vi "Open.vi"(8 "error in (no error)":errorcluster, 11 "DeploySerialResource in":refnum<class "SerialResource.lvclass">) -> (0 "error out":errorcluster, 3 "DeploySerialResource out":refnum<class "SerialResource.lvclass">)   [LabVIEW 2020, in "PicoG-Core.lvlib" / "SerialResource.lvclass"]
uses:
  SerialResource.lvclass
  SerialResource.lvclass/SerialResource.ctl
  <vilib>/IlluminatedG/IG Serial Stream/Stream-Serial/Serial Client/Serial Client.lvclass
  <vilib>/IlluminatedG/IG Serial Stream/Stream-Serial/Serial Client/Stop Bits.ctl
  <vilib>/IlluminatedG/IG Serial Stream/Stream-Serial/Serial Client/Flow Control.ctl
  <vilib>/IlluminatedG/IG Serial Stream/Stream-Serial/Serial Client/Parity.ctl
  <vilib>/IlluminatedG/IG Serial Stream/Stream-Serial/Serial Client/Port Config.ctl
  <vilib>/IlluminatedG/lv-stream/Endpoint/Endpoint.lvclass
  C:/Program Files (x86)/National Instruments/LabVIEW 2020/vi.lib/IlluminatedG/lv-stream/Connection/Connection.lvclass
  C:/Program Files (x86)/National Instruments/LabVIEW 2020/vi.lib/IlluminatedG/lv-stream/Endpoint/Endpoint.lvclass
  C:/Program Files (x86)/National Instruments/LabVIEW 2020/vi.lib/IlluminatedG/IG Serial Stream/Stream-Serial/Serial Client/Serial Client.lvclass
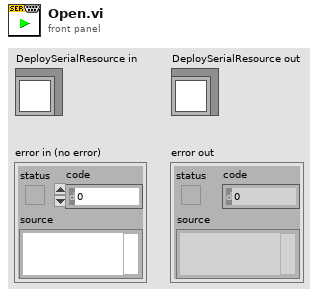
[diagram p1: front panel]
types:
  T1 = typedef "Stream-Serial.lvlib/Serial Client.lvclass/Port Config.ctl" = cluster{"Baud (115200)":u32, "Data Bits (8)":u8, "Stop Bits (1)":T2, "Flow Control":T3, "Use LineTerm?":bool, "LineTerm (\\n)":string, "Timeout ms (10000)":i32, "Parity (None)":T4}
  T2 = typedef "Stream-Serial.lvlib/Serial Client.lvclass/Stop Bits.ctl" = u16
  T3 = typedef "Stream-Serial.lvlib/Serial Client.lvclass/Flow Control.ctl" = u16
  T4 = typedef "Stream-Serial.lvlib/Serial Client.lvclass/Parity.ctl" = enum16{"None", "Odd", "Even", "Mark", "Space"}
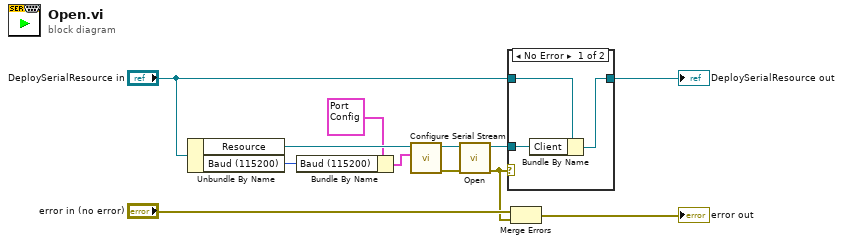
[diagram p0: block diagram]
diagram:
  n1 = Unbundle By Name("DeploySerialResource in") -> ("Resource"=w12:refnum<visa-resource-name>, "Baud (115200)"=w9:u32)
  n2 = Bundle By Name(cluster=T1 {"Baud (115200)"=115200, "Data Bits (8)"=8, "Stop Bits (1)"=10, "Flow Control"=0, "Use LineTerm?"=FALSE, "LineTerm (\\n)"="\n", "Timeout ms (10000)"=10000, "Parity (None)"=enum."None"} ("Port Config (115200 8N1)"), "Baud (115200)"=w9) -> (w10:T1)
  n3 = call <vilib>:"Configure Serial Stream.vi"("Port Config (115200 8N1)"=w10, "Serial Port"=w12) -> ("error out"=w6:errorcluster, "Serial Client out"=w7:refnum<class "Serial Client.lvclass">)  [unwired: 8 in]
  n4 = call <vilib>:"Open.vi"("error in (no error)"=w6, "Endpoint in"=w7) -> ("error out"=w1:errorcluster, "Endpoint out"=w5:refnum<class "Serial Client.lvclass">)  [unwired: 8 in]
  n5 = case shown="No Error" w1 {
    tunnel: "DeploySerialResource in" -> [w15 w16]
    tunnel: w5 -> [w14 _]
    tunnel: [w13 w16] -> w4
    frame No Error {
      n6 = Bundle By Name(cluster=w15, "Client"=w14) -> (w13:refnum<class "SerialResource.lvclass">)
    }
    frame Error {
    }
  }
  "DeploySerialResource out" <- w4
  n7 = Merge Errors("error in (no error)", w1) -> (→"error out":errorcluster)
